vi "Close.vi"(8 "error in":errorcluster, 11 "Cfg Dev in":refnum<class "Alicat Device.lvclass">) -> (0 "error out":errorcluster, 3 "Cfg Dev out":refnum<class "Alicat Device.lvclass">)   [LabVIEW 2015, in "Alicat Device.lvclass"]
uses:
  Alicat Device.lvclass
  Reusable/Session APIs/Text Communication/Text Device Session.lvclass
  Alicat Device.lvclass/Alicat Device.ctl
  Configurable Device/Configurable Device.lvclass
  <userlib>/_Session Fwk/Session - Root.lvclass
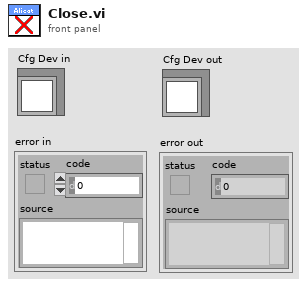
[diagram p1: front panel]
types:
  T1 = typedef "Session - Root.lvclass/Session Handle.ctl" = refnum<data-value>
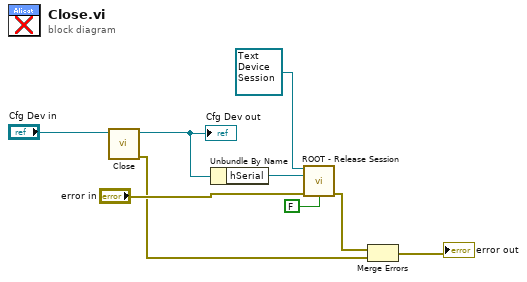
[diagram p0: block diagram]
diagram:
  n1 = call-parent "Close.vi"("Cfg Dev in"="Cfg Dev in") -> ("error out"=w1:errorcluster, "Cfg Dev out"=w2:refnum<class "Alicat Device.lvclass">)  [unwired: 9 in]
  "Cfg Dev out" <- w2
  n2 = Unbundle By Name(w2) -> ("hSerial"=w9:T1)
  n3 = call <userlib>:"ROOT - Release Session.vi"("OBJ - Session in"=refnum<class "Text Device Session.lvclass"> refnum ("Text Session"), "Session Handle in"=w9, "error in (no error)"="error in", "force destroy? (F)"=FALSE) -> ("error out"=w5:errorcluster)  [unwired: 10 in, 1 out]
  n4 = Merge Errors(w5, w1) -> (→"error out":errorcluster)
